vi "Calibrate_Gyro.vi"   [LabVIEW 2014]
uses:
  <userlib>/UCSD Robotics Lab/Robotics-Cape/LV/libroboticscape.lvlib
panel:
  # "Run this program to write new Gyro Calibration Values.  Keep BBB+Cape still during calibration routine"
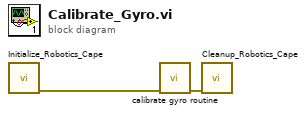
[diagram p0: block diagram]
diagram:
  n1 = call "Initialize_Robotics_Cape.vi"() -> ("error out"=w2:errorcluster)  [unwired: 11 in]
  n2 = call <userlib>:"calibrate gyro routine.vi"("error in (no error)"=w2) -> ("error out"=w1:errorcluster)  [unwired: 9 in, 1 out]
  n3 = call "Cleanup_Robotics_Cape.vi"("error in (no error)"=w1) -> ()  [unwired: 9 in, 2 out]
